vi "GLIMPSE Get region dimensions.vi"(11 "x1y1x2y2":u16[](array[numeric])) -> (0 "y size":u16, 1 "x size":u16, 2 "y origin":u16, 3 "x origin":u16)   [LabVIEW 2011]
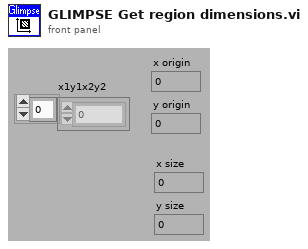
[diagram p1: front panel]
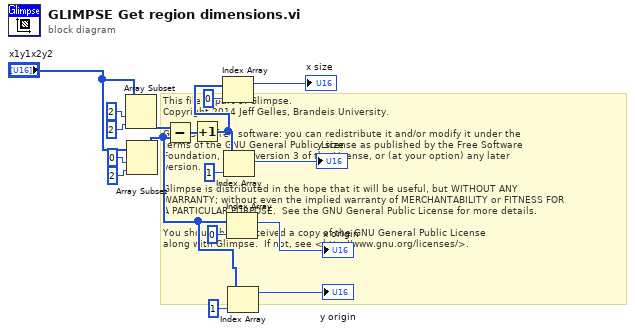
[diagram p0: block diagram]
diagram:
  # "This file is part of Glimpse. \nCopyright 2014 Jeff Gelles, Brandeis University.    \n\nGlimpse is free software: you can redistribute it and/or modify it under the \nterms of the GNU General Public License as published by the Free Software \nFoundation, either version 3 of the License, or (at your option) any later \nversion.\n\nGlimpse is distributed in the hope that it will be useful, but WITHOUT ANY \nWARRANTY; without even the implied warranty of MERCHANTABILITY or FITNESS FOR \nA PARTICULAR PURPOSE.  See the GNU General Public License for more details.\n\nYou should have received a copy of the GNU General Public License\nalong with Glimpse.  If not, see <http://www.gnu.org/licenses/>."
  n1 = Array Subset(array="x1y1x2y2", index=2, length=2) -> (w13:u16[])
  n2 = Array Subset(array="x1y1x2y2", index=0, length=2) -> (w3:u16[])
  n3 = Subtract(x=w13, y=w3) -> (x-y=w14:u16[])
  n4 = Increment(x=w14) -> (x+1=w15:u16[])
  n5 = Index Array(array=w15, index=0) -> (element=→"x size":u16)
  n6 = Index Array(array=w15, index=1) -> (element=→"y size":u16)
  n7 = Index Array(array=w3, index=0) -> (element=→"x origin":u16)
  n8 = Index Array(array=w3, index=1) -> (element=→"y origin":u16)
